vi "Actor Core.vi"(8 "error in":errorcluster, 11 "Nested in":refnum<class "Contador_Bin_Actor.lvclass">) -> (0 "error out":errorcluster, 3 "Actor out":refnum<class "Actor.lvclass">)   [LabVIEW 2019, in "Contador_Bin_Actor.lvlib" / "Contador_Bin_Actor.lvclass"]
doc: "(<B>Filename</B>: Actor Framework.lvlib:Actor.lvclass:Actor Core.vi)\n\nReceives messages to the actor, reacts to them, and initiates any error handling that may shut the actor down.\n\nDescendant classes may override this VI to append parallel tasks for the actor to complete while it handles messages. Overrides use the Call Parent Method node."
uses:
  Contador_Bin_Actor.lvclass
  C:/Program Files/National Instruments/LabVIEW 2019/vi.lib/ActorFramework/Actor/Actor.lvclass
  <vilib>/ActorFramework/Actor/Actor.lvclass
  Aumentar_contador/Aumentar_contador/Aumentar_contador.lvclass
  Logging_Contador_Actor/Logging_Contador_Actor/Logging_Contador_Actor.lvclass
  <vilib>/ActorFramework/Actor/Actor.lvclass/Actor.ctl
  <vilib>/ActorFramework/Message Enqueuer/Message Enqueuer.lvclass/Message Enqueuer.ctl
  Contador_Bin_Actor.lvclass/Contador_Bin_Actor.ctl
  Contador_Bin_Actor Messages/Start_Stop Msg/Start_Stop Msg.lvclass/Start_Stop Msg.ctl
  Contador_Bin_Actor Messages/Save_enable Msg/Save_enable Msg.lvclass/Save_enable Msg.ctl
  Contador_Bin_Actor Messages/File_path Msg/File_path Msg.lvclass/File_path Msg.ctl
  Contador_Bin_Actor Messages/C_format_file Msg/C_format_file Msg.lvclass/C_format_file Msg.ctl
  <vilib>/ActorFramework/Stop Msg/Stop Msg.lvclass/Stop Msg.ctl
  Contador_Bin_Actor Messages/Lim_Inf Msg/Lim_Inf Msg.lvclass/Lim_Inf Msg.ctl
  Contador_Bin_Actor Messages/Lim_Sup Msg/Lim_Sup Msg.lvclass/Lim_Sup Msg.ctl
  <vilib>/ActorFramework/Message Enqueuer/Init from Existing Queue.vi
  <vilib>/ActorFramework/Message Enqueuer/Enqueue.vi
  <vilib>/ActorFramework/Message Enqueuer/Enqueue Critical.vi
  Contador_Bin_Actor Messages/Start_Stop Msg/Start_Stop Msg.lvclass
  C:/Program Files/National Instruments/LabVIEW 2019/vi.lib/ActorFramework/Message/Message.lvclass
  Contador_Bin_Actor Messages/Save_enable Msg/Save_enable Msg.lvclass
  Contador_Bin_Actor Messages/File_path Msg/File_path Msg.lvclass
  Contador_Bin_Actor Messages/C_format_file Msg/C_format_file Msg.lvclass
  <vilib>/ActorFramework/Stop Msg/Stop Msg.lvclass
  Contador_Bin_Actor Messages/Lim_Inf Msg/Lim_Inf Msg.lvclass
  Contador_Bin_Actor Messages/Lim_Sup Msg/Lim_Sup Msg.lvclass
  <vilib>/ActorFramework/Message Priority Queue/Priority Enqueue.vi
  <vilib>/ActorFramework/Message Enqueuer/Message Enqueuer.lvclass
panel:
  out "Valor Decimal":u32
  out "Cuenta":bool[](array[boolean])
  in  "Format File":enum16{"TXT", "TDMS"}(ring)
  in  "Lim. Superior":u8
  in  "Lim. Inferior":u8
  in  "Exit":bool
  in  "Path":path
  in  "Save":bool
  in  "Stop":bool
  in  "Start":bool
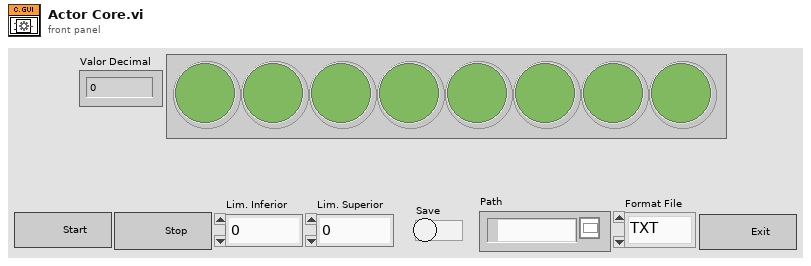
[diagram p1: front panel]
types:
  T1 = enum8{"Enabled", "Disabled", "Disabled and Grayed Out"}
  T2 = cluster{"Stop":refnum<user-event>, "Cuenta":refnum<user-event>}
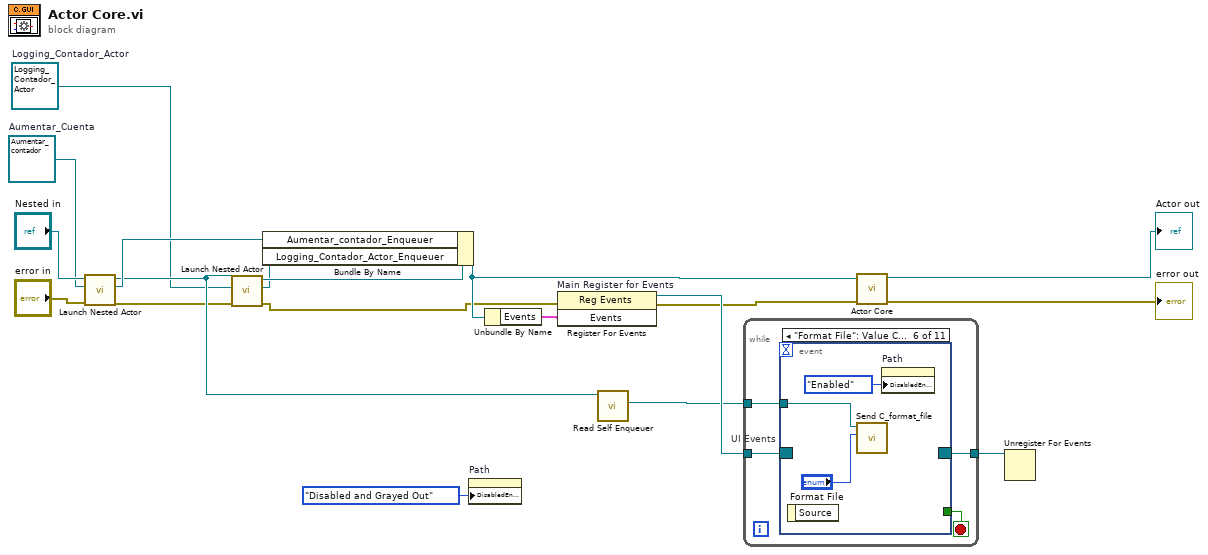
[diagram p0: block diagram]
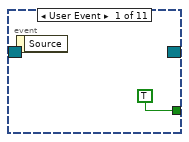
[diagram p2: hidden frame]
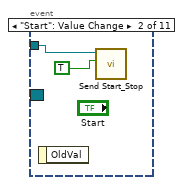
[diagram p3: hidden frame]
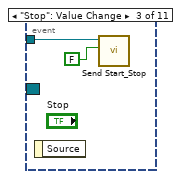
[diagram p4: hidden frame]
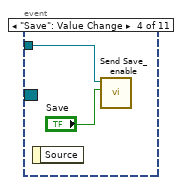
[diagram p5: hidden frame]
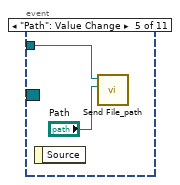
[diagram p6: hidden frame]
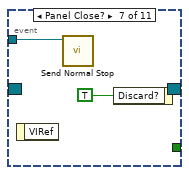
[diagram p7: hidden frame]
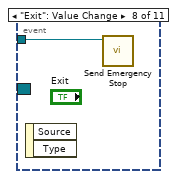
[diagram p8: hidden frame]
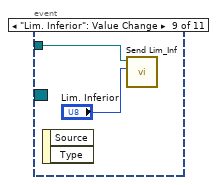
[diagram p9: hidden frame]
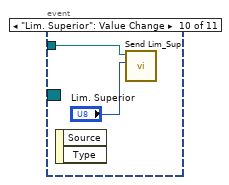
[diagram p10: hidden frame]
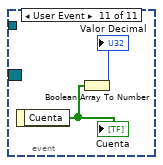
[diagram p11: hidden frame]
diagram:
  w5 = refnum<class "Logging_Contador_Actor.lvclass"> refnum  # Logging_Contador_Actor
  w10 = refnum<class "Aumentar_contador.lvclass"> refnum  # Aumentar_Cuenta
  n1 = call <vilib>:"Launch Nested Actor.vi"("error in (no error)"="error in", "Nested Actor"=w10, "Caller Actor in"="Nested in") -> ("error out"=w4:errorcluster, "Nested Actor's Enqueuer"=w9:refnum<class "Message Enqueuer.lvclass">, "Caller Actor out"=w6:refnum<class "Contador_Bin_Actor.lvclass">)  [unwired: 6 in]
  n2 = call <vilib>:"Launch Nested Actor.vi"("error in (no error)"=w4, "Nested Actor"=w5, "Caller Actor in"=w6) -> ("error out"=w3:errorcluster, "Nested Actor's Enqueuer"=w2:refnum<class "Message Enqueuer.lvclass">, "Caller Actor out"=w7:refnum<class "Contador_Bin_Actor.lvclass">)  [unwired: 6 in]
  n3 = Bundle By Name(cluster=w7, "Aumentar_contador_Enqueuer"=w9, "Logging_Contador_Actor_Enqueuer"=w2) -> (w8:refnum<class "Contador_Bin_Actor.lvclass">)
  n4 = property on="Path" class="Path"("DisabledEnum"=T1."Disabled and Grayed Out" ("Disabled")) -> ()  [unwired: 2 in, 2 out]
  n5 = Unbundle By Name(w8) -> ("Events"=w16:T2)
  n6 = register-events "Main Register for Events"(error in=w3, w16) -> (reference out=w17:refnum<event-registration>, error out=w12:errorcluster)  [unwired: 1 in]
  n7 = call <vilib>:"Read Self Enqueuer.vi"("Actor"=w6) -> ("Self Enqueuer"=w14:refnum<class "Message Enqueuer.lvclass">)  [unwired: 10 in]
  n8 = while {
    tunnel: w17 -> [w23]
    tunnel: [w21] -> w15
    tunnel: w14 -> [w20]
    stop <- w22 stop-if-true
    n9 = event "UI Events" shown="[5] \"Format File\": Value Change" {
      selector: w23 -> [_ _ _ _ _ _ _ _ _ _ _]
      dyn-events: [_ _ _ _ _ _ _ _ _ _ _] -> w21
      timeout: _ -> [_ _ _ _ _ _ _ _ _ _ _]
      tunnel: [TRUE _ _ _ _ _ _ _ _ _ _] -> w22
      tunnel: w20 -> [_ w26 w28 w30 w32 w35 w36 w38 w40 w42 _]
      event User Event {
        n10 = event-data() -> ()  [unwired: 1 in, 1 out]
      }
      event "Start": Value Change {
        n11 = event-data() -> ()  [unwired: 1 in, 1 out]
        n12 = call "Send Start_Stop.vi"("Start/Stop"=TRUE, "Message Enqueuer"=w26) -> ()  [unwired: 8 in, 2 out]
      }
      event "Stop": Value Change {
        n13 = event-data() -> ()  [unwired: 1 in, 1 out]
        n14 = call "Send Start_Stop.vi"("Start/Stop"=FALSE, "Message Enqueuer"=w28) -> ()  [unwired: 8 in, 2 out]
      }
      event "Save": Value Change {
        n15 = event-data() -> ()  [unwired: 1 in, 1 out]
        n16 = call "Send Save_enable.vi"("Save"="Save", "Message Enqueuer"=w30) -> ()  [unwired: 8 in, 2 out]
      }
      event "Path": Value Change {
        n17 = event-data() -> ()  [unwired: 1 in, 1 out]
        n18 = call "Send File_path.vi"("Path"="Path", "Message Enqueuer"=w32) -> ()  [unwired: 8 in, 2 out]
      }
      event "Format File": Value Change {
        n19 = event-data() -> ()  [unwired: 1 in, 1 out]
        n20 = call "Send C_format_file.vi"("Format File"="Format File", "Message Enqueuer"=w35) -> ()  [unwired: 8 in, 2 out]
        n21 = property on="Path" class="Path"("DisabledEnum"=T1."Enabled" ("Disabled")) -> ()  [unwired: 2 in, 2 out]
      }
      event Panel Close? {
        n22 = event-data() -> ()  [unwired: 1 in, 1 out]
        n23 = call <vilib>:"Send Normal Stop.vi"("Message Enqueuer"=w36) -> ()  [unwired: 10 in, 1 out]
        n24 = event-data("Discard?"=TRUE) -> ()  [unwired: 1 in, 1 out]
      }
      event "Exit": Value Change {
        n25 = event-data() -> ()  [unwired: 1 in, 2 out]
        n26 = call <vilib>:"Send Emergency Stop.vi"("Message Enqueuer"=w38) -> ()  [unwired: 10 in, 1 out]
      }
      event "Lim. Inferior": Value Change {
        n27 = event-data() -> ()  [unwired: 1 in, 2 out]
        n28 = call "Send Lim_Inf.vi"("Lim_Inf"="Lim. Inferior", "Message Enqueuer"=w40) -> ()  [unwired: 8 in, 2 out]
      }
      event "Lim. Superior": Value Change {
        n29 = event-data() -> ()  [unwired: 1 in, 2 out]
        n30 = call "Send Lim_Sup.vi"("Lim_Sup"="Lim. Superior", "Message Enqueuer"=w42) -> ()  [unwired: 8 in, 2 out]
      }
      event User Event {
        n31 = event-data() -> ("Cuenta"=w44:bool[])  [unwired: 1 in]
        "Cuenta" <- w44
        n32 = Boolean Array To Number(Boolean array=w44) -> (number=→"Valor Decimal":u32)
      }
    }
  }
  n33 = call-parent "Actor Core.vi"("error in"=w12, "Actor in"=w8) -> ("error out"=→"error out":errorcluster, "Actor out"=→"Actor out":refnum<class "Actor.lvclass">)  [unwired: 8 in]
  n34 = Unregister For Events(event registration refnum=w15) -> ()  [unwired: 1 in, 1 out]
